vi "五参数水样测试.vi"(11 "启动参数":T1={"测量模式"=enum."水样测试", "数据类型"="N", "手动启动标记"=FALSE, "测量时间"=3.0}) -> ()   [LabVIEW 2016, in "斯坦道多参数.lvlib"]
panel:
  out "Elapsed Time (s)":dbl caption="已用时间(s)"
  out "状态":string
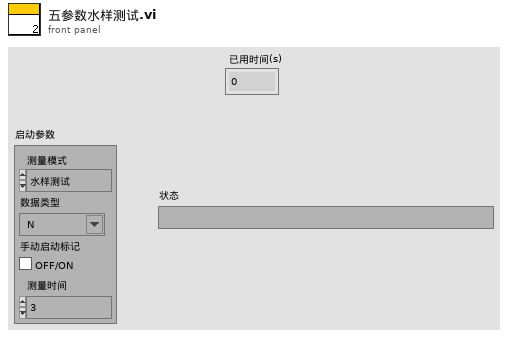
[diagram p1: front panel]
types:
  T1 = typedef "斯坦道多参数.lvlib/水样测试启动自定义输入参数.ctl" = cluster{"测量模式":enum16{"待机", "水样测试", "标样核查", "零点核查", "跨度核查", "空白测试", "平行样测试", "加标回收", "空白校准", "标样校准", "初始化（清洗）"}, "数据类型":string, "手动启动标记":bool, "测量时间":dbl}
  T2 = cluster{"时间标识":timestamp, "设备":string, "日志信息":string, "流程参数":string}
  T3 = cluster{"水温":bool, "pH":bool, "DO":bool, "DOper":bool, "电导率":bool, "ORP":bool, "浊度":bool, "叶绿素a":bool, "藻密度":bool}
  T4 = cluster{"水样数据时间":timestamp, "检测值":cluster{"水温":dbl, "pH":dbl, "DO":dbl, "DOper":dbl, "电导率":dbl, "ORP":dbl, "浊度":dbl, "叶绿素a":dbl, "藻密度":dbl}}
  T5 = cluster{"系统时间":timestamp, "工作状态":u16, "测量模式":u16, "告警代码":enum16{"无告警", "缺试剂告警", "缺水样告警", "缺蒸馏水告警", "缺标液告警", "仪表漏液告警", "标定异常告警", "超量程告警", "加热异常", "低试剂预警", "超上限告警", "超下限告警", "仪表内部其他异常", "滴定异常告警", "电极异常告警", "量程切换告警", "参数设置告警", "PH电极电位异常", "电导率电极异常", "浊度光度异常", "溶解氧电极异常", "溶解氧光强异常", "温度异常告警", "PH异常告警", "溶解氧异常告警", "电导率异常告警", "浊度异常告警", "叶绿素异常告警", "藻密度异常告警", "蓝绿藻异常告警", "ORP异常告警", "氨氮异常告警", "清洁刷异常告警", "SD卡异常告警", "蓝牙异常告警", "Wifi异常告警", "流程异常告警"}, "故障代码":enum16{"无故障", "电机故障", "温度故障", "通讯故障", "滴定故障"}, "日志代码":u16, "软件版本":string}
  T6 = cluster{"因子编码":string, "单位":string, "标样参考值":sgl, "水样数据时间":timestamp, "水样实测值":sgl, "水样数据标识":string, "K":sgl, "B":sgl, "T":sgl, "H":sgl, "水深":sgl, "探头温度":sgl}
  T7 = cluster{"水温":dbl, "pH":dbl, "DO":dbl, "Cond":dbl, "Turb":dbl, "叶绿素":dbl, "藻密度":dbl, "蓝绿藻":dbl, "ORP":dbl, "NH3N":dbl}
  T8 = enum16{"待机", "水样测试", "标样核查", "零点核查", "跨度核查", "空白测试", "平行样测试", "加标回收", "空白校准", "标样校准", "初始化（清洗）"}
  T9 = cluster{"数据类型":string, "测量模式":enum16{"待机", "水样测试", "标样核查", "零点核查", "跨度核查", "空白测试", "平行样测试", "加标回收", "空白校准", "标样校准", "初始化（清洗）"}, "database":string}
  T10 = cluster{"测量量程":dbl, "测量精度":dbl, "测量间隔":dbl, "消解温度":dbl, "消解时长":dbl, "空白校准时间":timestamp, "曲线截距":dbl, "曲线斜率":dbl, "测量检出限":dbl, "测量信号值":dbl, "线性相关系数":dbl, "二次多项式系数":dbl, "标样校准时间":timestamp, "稀释倍数":dbl, "三项式系数":dbl, "空白标定系数":dbl, "量程系数":dbl, "F0/ORPA":dbl, "F1/ORPB":dbl, "F2/ORPK":dbl, "F3":dbl, "F4":dbl, "F5":dbl, "F6":dbl, "F7":dbl, "X0/滴定数":dbl, "量程":dbl}
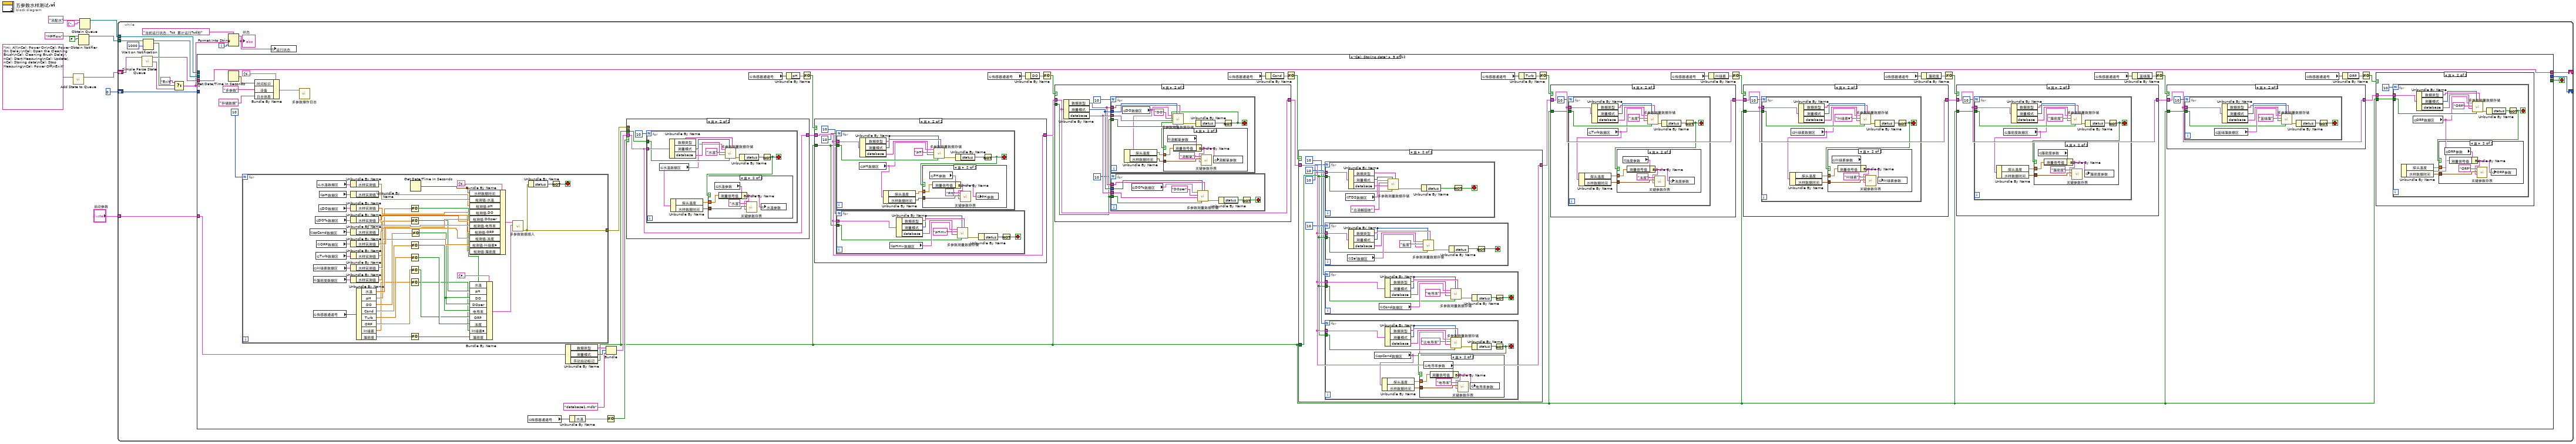
[diagram p0: block diagram]
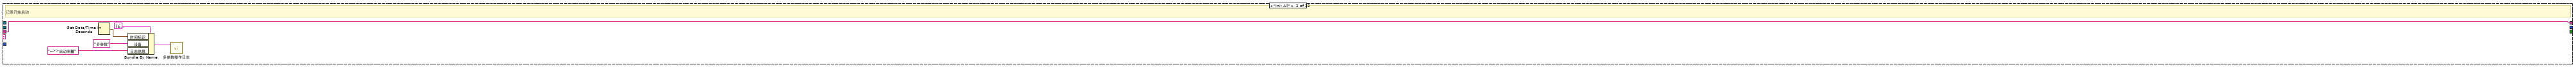
[diagram p3: hidden frame]
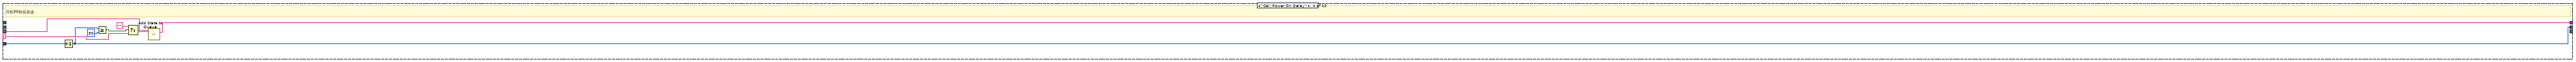
[diagram p5: hidden frame]
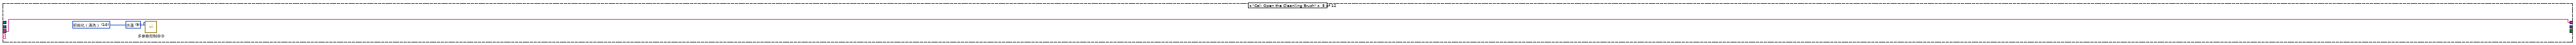
[diagram p6: hidden frame]
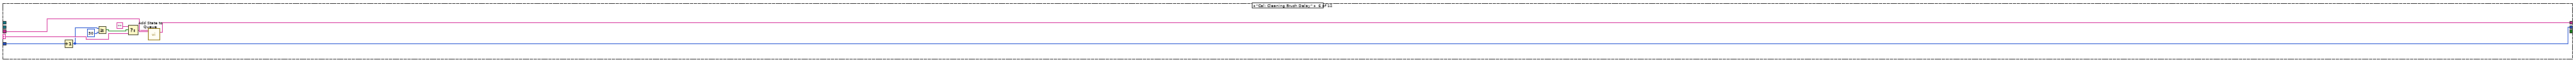
[diagram p7: hidden frame]
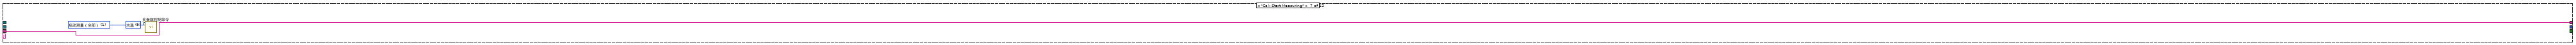
[diagram p8: hidden frame]
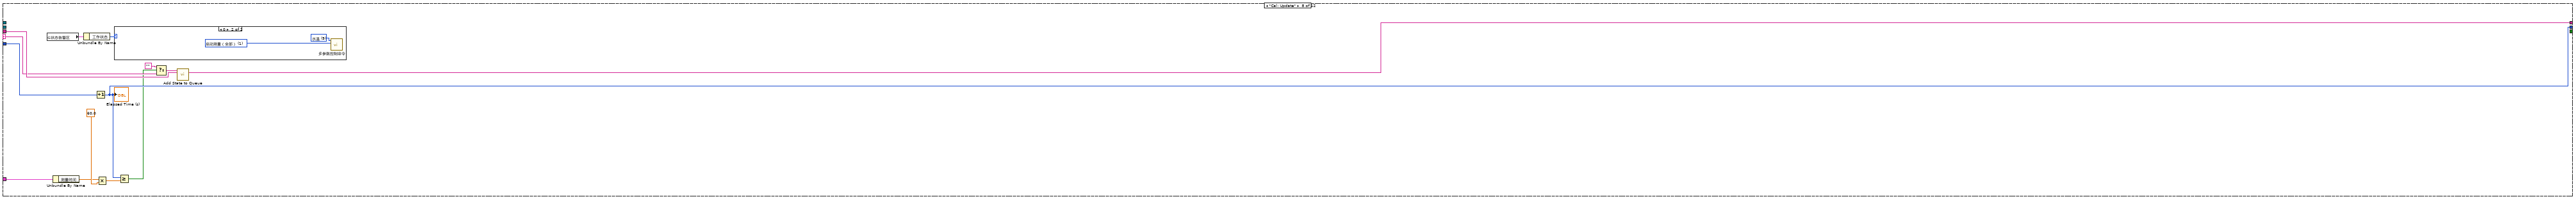
[diagram p9: hidden frame]
diagram:
  n1 = call "Add State to Queue.vi"("State(s) In (\"\")"="Ini: All\nCal: Power On\nCal: Power On Delay\nCal: Open the Cleaning Brush\nCal: Cleaning Brush Delay\nCal: Start Measuring\nCal: Update\nCal: Storing data\nCal: Stop Measuring\nCal: Power Off\nExit" ("State(s) In (\"\")")) -> ("States Out"=w9:string)  [unwired: 14 in]
  n2 = Obtain Notifier(name (unnamed)="MPFlow" ("名称（未命名）"), notification data type=FALSE) -> (notifier out=w3:refnum<notifier>)  [unwired: 2 in, 2 out]
  n3 = Obtain Queue(name (unnamed)="采配水" ("名称（未命名）"), element data type=cluster{"命令":string, "数据":variant} {"命令"="", "数据"=variant}) -> (queue out=w4:refnum<queue>)  [unwired: 3 in, 2 out]
  n4 = while {
    shift-right: [w26] -> _
    shift-left: w9 -> [w28]
    tunnel: w4 -> [w25]
    tunnel: w3 -> [w24]
    tunnel: "启动参数" -> [w23]
    shift-right: [w11] -> _
    shift-left: 0 -> [w12]
    i -> [w21]
    stop <- w19 stop-if-true
    n5 = call "Simple Parse State Queue.vi"("State Queue"=w28) -> ("Remain States"=w27:string, "Next State"=w14:string)  [unwired: 13 in]
    n6 = Wait on Notification(notifier=w24, timeout in ms (-1)=1000 ("超时毫秒(-1)")) -> (notifier out=w18:refnum<notifier>, notification=w16:bool)  [unwired: 2 in, 2 out]
    n7 = Select(t="Exit" ("State(s) In (\"\")"), s=w16, f=w14) -> (s? t:f=w13:string)
    n8 = case shown="\"Cal: Storing data\"" w13 {
      selector: w13 -> [_ _ _ w43 _ w53 _ w68 _ _ _ _]
      tunnel: w27 -> [w29 w35 w36 w45 w48 w57 w58 w69 w84 w406 w415 w418]
      tunnel: [w29 w35 w36 w44 w48 w56 w58 w65 w84 w406 w415 w418] -> w26
      tunnel: w25 -> [_ _ _ _ _ _ _ _ _ _ _ w417]
      tunnel: w18 -> [_ _ _ _ _ _ _ _ _ _ _ w416]
      tunnel: w23 -> [_ _ _ _ _ _ _ w70 w85 _ _ _]
      tunnel: [_ _ _ _ _ _ _ _ _ _ _ TRUE] -> w19
      tunnel: w12 -> [_ _ _ w40 _ w52 _ w64 _ _ _ _]
      tunnel: [_ _ _ w39 _ w51 _ w63 _ _ _ _] -> w11
      frame Default {
      }
      frame "Ini: All" {
        # "记录开始启动"
        n9 = Get Date/Time In Seconds() -> (seconds since 1Jan1904=w31:timestamp)
        n10 = Bundle By Name(cluster=T2 {"时间标识"=timestamp(0 s since 1904-01-01), "设备"="", "日志信息"="", "流程参数"=""} ("data in"), "时间标识"=w31, "设备"="多参数", "日志信息"="-->>启动测量") -> (w32:T2)
        n11 = call "多参数操作日志.vi"("data in"=w32) -> ()  [unwired: 10 in, 1 out]
      }
      frame "Cal: Power On" {
      }
      frame "Cal: Power On Delay" {
        # "开机30秒后发送"
        n12 = Increment(x=w40) -> (x+1=w39:i32)
        n13 = Greater Or Equal?(x=w39, y=30) -> (x >= y?=w37:bool)
        n14 = Select(t="", s=w37, f=w43) -> (s? t:f=w41:string)
        n15 = call "Add State to Queue.vi"("State(s) In Front (\"\")"=w41, "State(s) In (\"\")"=w45) -> ("States Out"=w44:string)  [unwired: 13 in]
      }
      frame "Cal: Open the Cleanling Brush" {
        w47 = u16 10 items=["启动测量（全部）"=1, "初始化（清洗）"=10, "停止测量（全部）"=11, "校时"=13, "启动测量（单个传感器）"=19, "停止测量（单个传感器）"=20] ("控制命令")
        w46 = u16 9 items=["氨氮"=3, "水温"=9, "pH值"=10, "溶解氧"=11, "电导率"=12, "浊度"=13, "叶绿素a"=14, "藻密度"=15, "蓝绿藻"=16, "氧化还原电位"=17, "溶解氧%"=18, "盐度"=19] ("站号")
        n16 = call "多参数控制命令.vi"("控制命令"=w47, "站号"=w46) -> ()  [unwired: 9 in, 1 out]
      }
      frame "Cal: Cleaning Brush Delay" {
        n17 = Increment(x=w52) -> (x+1=w51:i32)
        n18 = Greater Or Equal?(x=w51, y=30) -> (x >= y?=w49:bool)
        n19 = Select(t="", s=w49, f=w53) -> (s? t:f=w54:string)
        n20 = call "Add State to Queue.vi"("State(s) In Front (\"\")"=w54, "State(s) In (\"\")"=w57) -> ("States Out"=w56:string)  [unwired: 13 in]
      }
      frame "Cal: Start Measuring" {
        w60 = u16 1 items=["启动测量（全部）"=1, "初始化（清洗）"=10, "停止测量（全部）"=11, "校时"=13, "启动测量（单个传感器）"=19, "停止测量（单个传感器）"=20] ("控制命令")
        w59 = u16 9 items=["氨氮"=3, "水温"=9, "pH值"=10, "溶解氧"=11, "电导率"=12, "浊度"=13, "叶绿素a"=14, "藻密度"=15, "蓝绿藻"=16, "氧化还原电位"=17, "溶解氧%"=18, "盐度"=19] ("站号")
        n21 = call "多参数控制命令.vi"("控制命令"=w60, "站号"=w59) -> ()  [unwired: 9 in, 1 out]
      }
      frame "Cal: Update" {
        n22 = global read "多参数全局变量.vi" "状态告警区"() -> (w73:T5)
        n23 = Unbundle By Name(w70) -> ("测量时间"=w71:dbl)
        n24 = Unbundle By Name(w73) -> ("工作状态"=w74:u16)
        n25 = Increment(x=w64) -> (x+1=w63:i32)
        "Elapsed Time (s)" <- w63
        n26 = Multiply(x=w71, y=60.0) -> (x*y=w62:dbl)
        n27 = case shown="0" w74 {
          frame Default {
          }
          frame 0 {
            w75 = u16 1 items=["启动测量（全部）"=1, "初始化（清洗）"=10, "停止测量（全部）"=11, "校时"=13, "启动测量（单个传感器）"=19, "停止测量（单个传感器）"=20] ("控制命令")
            w76 = u16 9 items=["氨氮"=3, "水温"=9, "pH值"=10, "溶解氧"=11, "电导率"=12, "浊度"=13, "叶绿素a"=14, "藻密度"=15, "蓝绿藻"=16, "氧化还原电位"=17, "溶解氧%"=18, "盐度"=19] ("站号")
            n28 = call "多参数控制命令.vi"("控制命令"=w75, "站号"=w76) -> ()  [unwired: 9 in, 1 out]
          }
        }
        n29 = Greater Or Equal?(x=w63, y=w62) -> (x >= y?=w61:bool)
        n30 = Select(t="", s=w61, f=w68) -> (s? t:f=w67:string)
        n31 = call "Add State to Queue.vi"("State(s) In Front (\"\")"=w67, "State(s) In (\"\")"=w69) -> ("States Out"=w65:string)  [unwired: 13 in]
      }
      frame "Cal: Storing data" {
        n32 = Get Date/Time In Seconds() -> (seconds since 1Jan1904=w110:timestamp)
        n33 = for {
          N: 10 -> [_]
          tunnel: [w126] -> w77
          stop <- w127 stop-if-true
          n34 = global read "多参数全局变量.vi" "spCond数据区"() -> (w157:T6)
          n35 = global read "多参数全局变量.vi" "叶绿素数据区"() -> (w151:T6)
          n36 = global read "多参数全局变量.vi" "藻密度数据区"() -> (w149:T6)
          n37 = global read "多参数全局变量.vi" "传感器通道号"() -> (w143:T7)
          n38 = global read "多参数全局变量.vi" "DO%数据区"() -> (w159:T6)
          n39 = global read "多参数全局变量.vi" "Turb数据区"() -> (w153:T6)
          n40 = global read "多参数全局变量.vi" "ORP数据区"() -> (w155:T6)
          n41 = global read "多参数全局变量.vi" "水温数据区"() -> (w165:T6)
          n42 = global read "多参数全局变量.vi" "DO数据区"() -> (w161:T6)
          n43 = global read "多参数全局变量.vi" "pH数据区"() -> (w163:T6)
          n44 = Unbundle By Name(w165) -> ("水样实测值"=w164:sgl)
          n45 = Unbundle By Name(w163) -> ("水样实测值"=w162:sgl)
          n46 = Unbundle By Name(w161) -> ("水样实测值"=w160:sgl)
          n47 = Unbundle By Name(w159) -> ("水样实测值"=w158:sgl)
          n48 = Unbundle By Name(w157) -> ("水样实测值"=w156:sgl)
          n49 = Unbundle By Name(w155) -> ("水样实测值"=w154:sgl)
          n50 = Unbundle By Name(w153) -> ("水样实测值"=w152:sgl)
          n51 = Unbundle By Name(w151) -> ("水样实测值"=w150:sgl)
          n52 = Unbundle By Name(w149) -> ("水样实测值"=w148:sgl)
          n53 = Unbundle By Name(w143) -> ("水温"=w145:dbl, "pH"=w142:dbl, "DO"=w140:dbl, "Cond"=w138:dbl, "Turb"=w136:dbl, "ORP"=w134:dbl, "叶绿素"=w132:dbl, "藻密度"=w131:dbl)
          n54 = Not Equal To 0?(x=w145) -> (x != 0?=w144:bool)
          n55 = Not Equal To 0?(x=w142) -> (x != 0?=w141:bool)
          n56 = Not Equal To 0?(x=w138) -> (x != 0?=w137:bool)
          n57 = Not Equal To 0?(x=w136) -> (x != 0?=w135:bool)
          n58 = Not Equal To 0?(x=w134) -> (x != 0?=w133:bool)
          n59 = Not Equal To 0?(x=w132) -> (x != 0?=w130:bool)
          n60 = Not Equal To 0?(x=w131) -> (x != 0?=w129:bool)
          n61 = Get Date/Time In Seconds() -> (seconds since 1Jan1904=w166:timestamp)
          n62 = Not Equal To 0?(x=w140) -> (x != 0?=w139:bool)
          n63 = Bundle By Name(cluster=T4 {"水样数据时间"=timestamp(0 s since 1904-01-01), "检测值"={"水温"=0.0, "pH"=0.0, "DO"=0.0, "DOper"=0.0, "电导率"=0.0, "ORP"=0.0, "浊度"=0.0, "叶绿素a"=0.0, "藻密度"=0.0}} ("data in"), "水样数据时间"=w166, "检测值.水温"=w164, "检测值.pH"=w162, "检测值.DO"=w160, "检测值.DOper"=w158, "检测值.电导率"=w156, "检测值.ORP"=w154, "检测值.浊度"=w152, "检测值.叶绿素a"=w150, "检测值.藻密度"=w148) -> (w167:T4)
          n64 = Bundle By Name(cluster=T3 {"水温"=FALSE, "pH"=FALSE, "DO"=FALSE, "DOper"=FALSE, "电导率"=FALSE, "ORP"=FALSE, "浊度"=FALSE, "叶绿素a"=FALSE, "藻密度"=FALSE} ("columns enable"), "水温"=w144, "pH"=w141, "DO"=w139, "DOper"=w139, "电导率"=w137, "ORP"=w133, "浊度"=w135, "叶绿素a"=w130, "藻密度"=w129) -> (w146:T3)
          n65 = call "多参数数据插入.vi"("columns enable"=w146, "data in"=w167) -> ("error out"=w126:errorcluster)  [unwired: 9 in]
          n66 = Unbundle By Name(w126) -> ("status"=w128:bool)
          n67 = Not(x=w128) -> (.not. x?=w127:bool)
        }
        n68 = Bundle By Name(cluster=T2 {"时间标识"=timestamp(0 s since 1904-01-01), "设备"="", "日志信息"="", "流程参数"=""} ("data in"), "时间标识"=w110, "设备"="多参数", "日志信息"="存储数据") -> (w111:T2)
        n69 = call "多参数操作日志.vi"("data in"=w111) -> ()  [unwired: 10 in, 1 out]
        n70 = global read "多参数全局变量.vi" "传感器通道号"() -> (w86:T7)
        n71 = Unbundle By Name(w85) -> ("数据类型"=w102:string, "测量模式"=w103:T8, "手动启动标记"=w79:bool)
        n72 = Unbundle By Name(w86) -> ("水温"=w87:dbl)
        n73 = Not Equal To 0?(x=w87) -> (x != 0?=w88:bool)
        n74 = Bundle("数据类型"=w102, "测量模式"=w103, "database"="database1.mdb") -> (w104:T9)  [unwired: 1 in]
        n75 = case shown="真" w88 {
          tunnel: w104 -> [w385 w388]
          tunnel: [w385 w388] -> w105
          tunnel: w79 -> [_ w387]
          tunnel: w77 -> [_ _]
          frame False {
          }
          frame True {
            n76 = for {
              N: 10 -> [_]
              tunnel: w388 -> [w399]
              tunnel: w387 -> [w395]
              stop <- w389 stop-if-true
              n77 = global read "多参数全局变量.vi" "水温数据区"() -> (w392:T6)
              n78 = Unbundle By Name(w399) -> ("数据类型"=w398:string, "测量模式"=w397:T8, "database"=w396:string)
              n79 = Unbundle By Name(w392) -> ("探头温度"=w390:sgl, "水样数据时间"=w391:timestamp)
              n80 = call "多参数测量数据存储.vi"("数据类型"=w398, "手动启动标记"=w395, "测量模式"=w397, "database"=w396, "table输入"="水温", "data in"=w392) -> ("error out"=w394:errorcluster)  [unwired: 5 in]
              n81 = Unbundle By Name(w394) -> ("status"=w393:bool)
              n82 = Not(x=w393) -> (.not. x?=w389:bool)
              n83 = case shown="真" w389 {
                tunnel: w391 -> [_ w403]
                tunnel: w390 -> [_ w402]
                frame False {
                }
                frame True {
                  n84 = global read "多参数断电保存全局变量.vi" "水温参数"() -> (w405:T10)
                  n85 = Bundle By Name(cluster=w405, "测量信号值"=w402) -> (w401:T10)
                  n86 = call "关键参数存表.vi"("仪器参数"=w401, "datatime"=w403, "仪器名称"="水温") -> ()  [unwired: 8 in, 1 out]
                  n87 = global write "多参数断电保存全局变量.vi" "水温参数"(w401) -> ()
                }
              }
            }
          }
        }
        n88 = global read "多参数全局变量.vi" "传感器通道号"() -> (w93:T7)
        n89 = Unbundle By Name(w93) -> ("pH"=w94:dbl)
        n90 = Not Equal To 0?(x=w94) -> (x != 0?=w89:bool)
        n91 = case shown="真" w89 {
          tunnel: w105 -> [w353 w357]
          tunnel: [w353 w357] -> w107
          tunnel: w79 -> [_ w355]
          frame False {
          }
          frame True {
            n92 = for {
              N: 10 -> [_]
              tunnel: w357 -> [w375]
              tunnel: w355 -> [w373]
              stop <- w371 stop-if-true
              n93 = global read "多参数全局变量.vi" "pH数据区"() -> (w370:T6)
              n94 = Unbundle By Name(w375) -> ("数据类型"=w378:string, "测量模式"=w377:T8, "database"=w376:string)
              n95 = Unbundle By Name(w370) -> ("探头温度"=w369:sgl, "水样数据时间"=w368:timestamp)
              n96 = call "多参数测量数据存储.vi"("数据类型"=w378, "手动启动标记"=w373, "测量模式"=w377, "database"=w376, "table输入"="pH", "data in"=w370) -> ("error out"=w374:errorcluster)  [unwired: 5 in]
              n97 = Unbundle By Name(w374) -> ("status"=w372:bool)
              n98 = Not(x=w372) -> (.not. x?=w371:bool)
              n99 = case shown="真" w371 {
                tunnel: w368 -> [_ w382]
                tunnel: w369 -> [_ w381]
                frame False {
                }
                frame True {
                  n100 = global read "多参数断电保存全局变量.vi" "PH参数"() -> (w384:T10)
                  n101 = Bundle By Name(cluster=w384, "测量信号值"=w381) -> (w380:T10)
                  n102 = call "关键参数存表.vi"("仪器参数"=w380, "datatime"=w382, "仪器名称"="PH") -> ()  [unwired: 8 in, 1 out]
                  n103 = global write "多参数断电保存全局变量.vi" "PH参数"(w380) -> ()
                }
              }
            }
            n104 = for {
              N: 10 -> [_]
              tunnel: w357 -> [w367]
              tunnel: w355 -> [w361]
              stop <- w358 stop-if-true
              n105 = global read "多参数全局变量.vi" "pHmv数据区"() -> (w363:T6)
              n106 = Unbundle By Name(w367) -> ("数据类型"=w366:string, "测量模式"=w365:T8, "database"=w364:string)
              n107 = call "多参数测量数据存储.vi"("数据类型"=w366, "手动启动标记"=w361, "测量模式"=w365, "database"=w364, "table输入"="pHmv", "data in"=w363) -> ("error out"=w360:errorcluster)  [unwired: 5 in]
              n108 = Unbundle By Name(w360) -> ("status"=w359:bool)
              n109 = Not(x=w359) -> (.not. x?=w358:bool)
            }
          }
        }
        n110 = global read "多参数全局变量.vi" "传感器通道号"() -> (w95:T7)
        n111 = Unbundle By Name(w95) -> ("DO"=w96:dbl)
        n112 = Not Equal To 0?(x=w96) -> (x != 0?=w90:bool)
        n113 = case shown="真" w90 {
          tunnel: [w320 w327] -> w106
          tunnel: w107 -> [w320 w327]
          tunnel: w79 -> [_ w323]
          frame False {
          }
          frame True {
            n114 = Unbundle By Name(w327) -> ("数据类型"=w324:string, "测量模式"=w325:T8, "database"=w326:string)
            n115 = for {
              N: 10 -> [_]
              tunnel: w326 -> [w337]
              tunnel: w325 -> [w336]
              tunnel: w324 -> [w335]
              tunnel: w323 -> [w334]
              stop <- w331 stop-if-true
              n116 = global read "多参数全局变量.vi" "DO数据区"() -> (w330:T6)
              n117 = Unbundle By Name(w330) -> ("探头温度"=w328:sgl, "水样数据时间"=w329:timestamp)
              n118 = call "多参数测量数据存储.vi"("数据类型"=w335, "手动启动标记"=w334, "测量模式"=w336, "database"=w337, "table输入"="DO", "data in"=w330) -> ("error out"=w333:errorcluster)  [unwired: 5 in]
              n119 = Unbundle By Name(w333) -> ("status"=w332:bool)
              n120 = Not(x=w332) -> (.not. x?=w331:bool)
              n121 = case shown="真" w331 {
                tunnel: w329 -> [_ w341]
                tunnel: w328 -> [_ w340]
                frame False {
                }
                frame True {
                  n122 = global read "多参数断电保存全局变量.vi" "溶解氧参数"() -> (w343:T10)
                  n123 = Bundle By Name(cluster=w343, "测量信号值"=w340) -> (w339:T10)
                  n124 = call "关键参数存表.vi"("仪器参数"=w339, "datatime"=w341, "仪器名称"="溶解氧") -> ()  [unwired: 8 in, 1 out]
                  n125 = global write "多参数断电保存全局变量.vi" "溶解氧参数"(w339) -> ()
                }
              }
            }
            n126 = for {
              N: 10 -> [_]
              tunnel: w326 -> [w350]
              tunnel: w325 -> [w349]
              tunnel: w324 -> [w348]
              tunnel: w323 -> [w347]
              stop <- w344 stop-if-true
              n127 = global read "多参数全局变量.vi" "DO%数据区"() -> (w352:T6)
              n128 = call "多参数测量数据存储.vi"("数据类型"=w348, "手动启动标记"=w347, "测量模式"=w349, "database"=w350, "table输入"="DOper", "data in"=w352) -> ("error out"=w346:errorcluster)  [unwired: 5 in]
              n129 = Unbundle By Name(w346) -> ("status"=w345:bool)
              n130 = Not(x=w345) -> (.not. x?=w344:bool)
            }
          }
        }
        n131 = global read "多参数全局变量.vi" "传感器通道号"() -> (w97:T7)
        n132 = Unbundle By Name(w97) -> ("Cond"=w98:dbl)
        n133 = Not Equal To 0?(x=w98) -> (x != 0?=w91:bool)
        n134 = case shown="真" w91 {
          tunnel: w106 -> [w266 w272]
          tunnel: [w266 w272] -> w108
          tunnel: w79 -> [_ w271]
          frame False {
          }
          frame True {
            n135 = for {
              N: 10 -> [_]
              tunnel: w272 -> [w282]
              tunnel: w271 -> [w276]
              stop <- w273 stop-if-true
              n136 = global read "多参数全局变量.vi" "TDS数据区"() -> (w278:T6)
              n137 = Unbundle By Name(w282) -> ("数据类型"=w279:string, "测量模式"=w280:T8, "database"=w281:string)
              n138 = call "多参数测量数据存储.vi"("数据类型"=w279, "手动启动标记"=w276, "测量模式"=w280, "database"=w281, "table输入"="总溶解固体", "data in"=w278) -> ("error out"=w275:errorcluster)  [unwired: 5 in]
              n139 = Unbundle By Name(w275) -> ("status"=w274:bool)
              n140 = Not(x=w274) -> (.not. x?=w273:bool)
            }
            n141 = for {
              N: 10 -> [_]
              tunnel: w272 -> [w304]
              tunnel: w271 -> [w303]
              stop <- w300 stop-if-true
              n142 = global read "多参数全局变量.vi" "Sal数据区"() -> (w309:T6)
              n143 = Unbundle By Name(w304) -> ("数据类型"=w307:string, "测量模式"=w306:T8, "database"=w305:string)
              n144 = call "多参数测量数据存储.vi"("数据类型"=w307, "手动启动标记"=w303, "测量模式"=w306, "database"=w305, "table输入"="盐度", "data in"=w309) -> ("error out"=w302:errorcluster)  [unwired: 5 in]
              n145 = Unbundle By Name(w302) -> ("status"=w301:bool)
              n146 = Not(x=w301) -> (.not. x?=w300:bool)
            }
            n147 = for {
              N: 10 -> [_]
              tunnel: w272 -> [w314]
              tunnel: w271 -> [w313]
              stop <- w310 stop-if-true
              n148 = global read "多参数全局变量.vi" "Cond数据区"() -> (w319:T6)
              n149 = Unbundle By Name(w314) -> ("数据类型"=w316:string, "测量模式"=w315:T8, "database"=w317:string)
              n150 = call "多参数测量数据存储.vi"("数据类型"=w316, "手动启动标记"=w313, "测量模式"=w315, "database"=w317, "table输入"="电导率", "data in"=w319) -> ("error out"=w312:errorcluster)  [unwired: 5 in]
              n151 = Unbundle By Name(w312) -> ("status"=w311:bool)
              n152 = Not(x=w311) -> (.not. x?=w310:bool)
            }
            n153 = for {
              N: 10 -> [_]
              tunnel: w272 -> [w294]
              tunnel: w271 -> [w289]
              stop <- w284 stop-if-true
              n154 = global read "多参数全局变量.vi" "spCond数据区"() -> (w283:T6)
              n155 = Unbundle By Name(w283) -> ("探头温度"=w285:sgl, "水样数据时间"=w286:timestamp)
              n156 = Unbundle By Name(w294) -> ("数据类型"=w293:string, "测量模式"=w292:T8, "database"=w291:string)
              n157 = call "多参数测量数据存储.vi"("数据类型"=w293, "手动启动标记"=w289, "测量模式"=w292, "database"=w291, "table输入"="比电导率", "data in"=w283) -> ("error out"=w288:errorcluster)  [unwired: 5 in]
              n158 = Unbundle By Name(w288) -> ("status"=w287:bool)
              n159 = Not(x=w287) -> (.not. x?=w284:bool)
              n160 = case shown="真" w284 {
                tunnel: w286 -> [_ w297]
                tunnel: w285 -> [_ w296]
                frame False {
                }
                frame True {
                  n161 = global read "多参数断电保存全局变量.vi" "电导率参数"() -> (w299:T10)
                  n162 = Bundle By Name(cluster=w299, "测量信号值"=w296) -> (w295:T10)
                  n163 = call "关键参数存表.vi"("仪器参数"=w295, "datatime"=w297, "仪器名称"="电导率") -> ()  [unwired: 8 in, 1 out]
                  n164 = global write "多参数断电保存全局变量.vi" "电导率参数"(w295) -> ()
                }
              }
            }
          }
        }
        n165 = global read "多参数全局变量.vi" "传感器通道号"() -> (w99:T7)
        n166 = Unbundle By Name(w99) -> ("Turb"=w100:dbl)
        n167 = Not Equal To 0?(x=w100) -> (x != 0?=w92:bool)
        n168 = case shown="真" w92 {
          tunnel: w108 -> [w245 w248]
          tunnel: [w245 w248] -> w117
          tunnel: w79 -> [_ w247]
          frame False {
          }
          frame True {
            n169 = for {
              N: 10 -> [_]
              tunnel: w248 -> [w256]
              tunnel: w247 -> [w255]
              stop <- w249 stop-if-true
              n170 = global read "多参数全局变量.vi" "Turb数据区"() -> (w250:T6)
              n171 = Unbundle By Name(w250) -> ("探头温度"=w251:sgl, "水样数据时间"=w252:timestamp)
              n172 = Unbundle By Name(w256) -> ("数据类型"=w257:string, "测量模式"=w258:T8, "database"=w259:string)
              n173 = call "多参数测量数据存储.vi"("数据类型"=w257, "手动启动标记"=w255, "测量模式"=w258, "database"=w259, "table输入"="浊度", "data in"=w250) -> ("error out"=w254:errorcluster)  [unwired: 5 in]
              n174 = Unbundle By Name(w254) -> ("status"=w253:bool)
              n175 = Not(x=w253) -> (.not. x?=w249:bool)
              n176 = case shown="真" w249 {
                tunnel: w252 -> [_ w263]
                tunnel: w251 -> [_ w262]
                frame False {
                }
                frame True {
                  n177 = global read "多参数断电保存全局变量.vi" "浊度参数"() -> (w265:T10)
                  n178 = Bundle By Name(cluster=w265, "测量信号值"=w262) -> (w261:T10)
                  n179 = call "关键参数存表.vi"("仪器参数"=w261, "datatime"=w263, "仪器名称"="浊度") -> ()  [unwired: 8 in, 1 out]
                  n180 = global write "多参数断电保存全局变量.vi" "浊度参数"(w261) -> ()
                }
              }
            }
          }
        }
        n181 = global read "多参数全局变量.vi" "传感器通道号"() -> (w115:T7)
        n182 = Unbundle By Name(w115) -> ("叶绿素"=w114:dbl)
        n183 = Not Equal To 0?(x=w114) -> (x != 0?=w116:bool)
        n184 = case shown="真" w116 {
          tunnel: w117 -> [w224 w227]
          tunnel: [w224 w227] -> w121
          tunnel: w79 -> [_ w226]
          frame False {
          }
          frame True {
            n185 = for {
              N: 10 -> [_]
              tunnel: w227 -> [w235]
              tunnel: w226 -> [w234]
              stop <- w229 stop-if-true
              n186 = global read "多参数全局变量.vi" "叶绿素数据区"() -> (w228:T6)
              n187 = Unbundle By Name(w228) -> ("探头温度"=w230:sgl, "水样数据时间"=w231:timestamp)
              n188 = Unbundle By Name(w235) -> ("数据类型"=w236:string, "测量模式"=w237:T8, "database"=w238:string)
              n189 = call "多参数测量数据存储.vi"("数据类型"=w236, "手动启动标记"=w234, "测量模式"=w237, "database"=w238, "table输入"="叶绿素a", "data in"=w228) -> ("error out"=w233:errorcluster)  [unwired: 5 in]
              n190 = Unbundle By Name(w233) -> ("status"=w232:bool)
              n191 = Not(x=w232) -> (.not. x?=w229:bool)
              n192 = case shown="真" w229 {
                tunnel: w231 -> [_ w242]
                tunnel: w230 -> [_ w241]
                frame False {
                }
                frame True {
                  n193 = global read "多参数断电保存全局变量.vi" "叶绿素参数"() -> (w244:T10)
                  n194 = Bundle By Name(cluster=w244, "测量信号值"=w241) -> (w240:T10)
                  n195 = call "关键参数存表.vi"("仪器参数"=w240, "datatime"=w242, "仪器名称"="叶绿素") -> ()  [unwired: 8 in, 1 out]
                  n196 = global write "多参数断电保存全局变量.vi" "叶绿素参数"(w240) -> ()
                }
              }
            }
          }
        }
        n197 = global read "多参数全局变量.vi" "传感器通道号"() -> (w119:T7)
        n198 = Unbundle By Name(w119) -> ("藻密度"=w120:dbl)
        n199 = Not Equal To 0?(x=w120) -> (x != 0?=w118:bool)
        n200 = case shown="真" w118 {
          tunnel: w121 -> [w203 w206]
          tunnel: [w203 w206] -> w125
          tunnel: w79 -> [_ w205]
          frame False {
          }
          frame True {
            n201 = for {
              N: 10 -> [_]
              tunnel: w206 -> [w214]
              tunnel: w205 -> [w213]
              stop <- w208 stop-if-true
              n202 = global read "多参数全局变量.vi" "藻密度数据区"() -> (w207:T6)
              n203 = Unbundle By Name(w207) -> ("探头温度"=w209:sgl, "水样数据时间"=w210:timestamp)
              n204 = Unbundle By Name(w214) -> ("数据类型"=w215:string, "测量模式"=w216:T8, "database"=w217:string)
              n205 = call "多参数测量数据存储.vi"("数据类型"=w215, "手动启动标记"=w213, "测量模式"=w216, "database"=w217, "table输入"="藻密度", "data in"=w207) -> ("error out"=w212:errorcluster)  [unwired: 5 in]
              n206 = Unbundle By Name(w212) -> ("status"=w211:bool)
              n207 = Not(x=w211) -> (.not. x?=w208:bool)
              n208 = case shown="真" w208 {
                tunnel: w210 -> [_ w221]
                tunnel: w209 -> [_ w220]
                frame False {
                }
                frame True {
                  n209 = global read "多参数断电保存全局变量.vi" "藻密度参数"() -> (w223:T10)
                  n210 = Bundle By Name(cluster=w223, "测量信号值"=w220) -> (w219:T10)
                  n211 = call "关键参数存表.vi"("仪器参数"=w219, "datatime"=w221, "仪器名称"="藻密度") -> ()  [unwired: 8 in, 1 out]
                  n212 = global write "多参数断电保存全局变量.vi" "藻密度参数"(w219) -> ()
                }
              }
            }
          }
        }
        n213 = global read "多参数全局变量.vi" "传感器通道号"() -> (w123:T7)
        n214 = Unbundle By Name(w123) -> ("蓝绿藻"=w122:dbl)
        n215 = Not Equal To 0?(x=w122) -> (x != 0?=w124:bool)
        n216 = case shown="真" w124 {
          tunnel: w125 -> [w189 w190]
          tunnel: w79 -> [_ w192]
          tunnel: [w189 w190] -> w83
          frame False {
          }
          frame True {
            n217 = for {
              N: 10 -> [_]
              tunnel: w190 -> [w200]
              tunnel: w192 -> [w196]
              stop <- w193 stop-if-true
              n218 = global read "多参数全局变量.vi" "蓝绿藻数据区"() -> (w202:T6)
              n219 = Unbundle By Name(w200) -> ("数据类型"=w197:string, "测量模式"=w198:T8, "database"=w199:string)
              n220 = call "多参数测量数据存储.vi"("数据类型"=w197, "手动启动标记"=w196, "测量模式"=w198, "database"=w199, "table输入"="蓝绿藻", "data in"=w202) -> ("error out"=w195:errorcluster)  [unwired: 5 in]
              n221 = Unbundle By Name(w195) -> ("status"=w194:bool)
              n222 = Not(x=w194) -> (.not. x?=w193:bool)
            }
          }
        }
        n223 = global read "多参数全局变量.vi" "传感器通道号"() -> (w81:T7)
        n224 = Unbundle By Name(w81) -> ("ORP"=w82:dbl)
        n225 = Not Equal To 0?(x=w82) -> (x != 0?=w80:bool)
        n226 = case shown="真" w80 {
          tunnel: w83 -> [_ w171]
          tunnel: w79 -> [_ w170]
          frame False {
          }
          frame True {
            n227 = for {
              N: 10 -> [_]
              tunnel: w171 -> [w182]
              tunnel: w170 -> [w178]
              stop <- w173 stop-if-true
              n228 = global read "多参数全局变量.vi" "ORP数据区"() -> (w172:T6)
              n229 = Unbundle By Name(w172) -> ("探头温度"=w174:sgl, "水样数据时间"=w175:timestamp)
              n230 = Unbundle By Name(w182) -> ("数据类型"=w179:string, "测量模式"=w180:T8, "database"=w181:string)
              n231 = call "多参数测量数据存储.vi"("数据类型"=w179, "手动启动标记"=w178, "测量模式"=w180, "database"=w181, "table输入"="ORP", "data in"=w172) -> ("error out"=w177:errorcluster)  [unwired: 5 in]
              n232 = Unbundle By Name(w177) -> ("status"=w176:bool)
              n233 = Not(x=w176) -> (.not. x?=w173:bool)
              n234 = case shown="真" w173 {
                tunnel: w175 -> [_ w186]
                tunnel: w174 -> [_ w185]
                frame False {
                }
                frame True {
                  n235 = global read "多参数断电保存全局变量.vi" "ORP参数"() -> (w188:T10)
                  n236 = Bundle By Name(cluster=w188, "测量信号值"=w185) -> (w184:T10)
                  n237 = call "关键参数存表.vi"("仪器参数"=w184, "datatime"=w186, "仪器名称"="ORP") -> ()  [unwired: 8 in, 1 out]
                  n238 = global write "多参数断电保存全局变量.vi" "ORP参数"(w184) -> ()
                }
              }
            }
          }
        }
      }
      frame "Cal: Stop Measuring" {
        n239 = flat-sequence {
          frame #0 {
            w412 = u16 11 items=["启动测量（全部）"=1, "初始化（清洗）"=10, "停止测量（全部）"=11, "校时"=13, "启动测量（单个传感器）"=19, "停止测量（单个传感器）"=20] ("控制命令")
            w413 = u16 9 items=["氨氮"=3, "水温"=9, "pH值"=10, "溶解氧"=11, "电导率"=12, "浊度"=13, "叶绿素a"=14, "藻密度"=15, "蓝绿藻"=16, "氧化还原电位"=17, "溶解氧%"=18, "盐度"=19] ("站号")
            n240 = call "多参数控制命令.vi"("控制命令"=w412, "站号"=w413) -> ()  [unwired: 9 in, 1 out]
          }
          frame #1 {
            n241 = Wait (ms)(milliseconds to wait=u32 2000 ("等待时间（毫秒）")) -> ()  [unwired: 1 out]
          }
        }
        n242 = Get Date/Time In Seconds() -> (seconds since 1Jan1904=w409:timestamp)
        n243 = Bundle By Name(cluster=T2 {"时间标识"=timestamp(0 s since 1904-01-01), "设备"="", "日志信息"="", "流程参数"=""} ("data in"), "时间标识"=w409, "设备"="多参数", "日志信息"="-->>停止测量") -> (w408:T2)
        n244 = call "多参数操作日志.vi"("data in"=w408) -> ()  [unwired: 10 in, 1 out]
      }
      frame "Cal: Power Off" {
      }
      frame "Exit" {
        n245 = Release Queue(queue=w417) -> ()  [unwired: 2 in, 3 out]
        n246 = Release Notifier(notifier=w416) -> ()  [unwired: 2 in, 3 out]
      }
    }
    n247 = Format Into String(format string="当前运行状态：%s  累计运行%d秒" ("格式字符串"), w13, w21) -> (resulting string=w20:string)  [unwired: 2 in, 1 out]
    "状态" <- w20
    n248 = global write "多参数全局变量.vi" "运行状态"(w20) -> ()
  }
